vi "QPSK Modulation.vi"(10 "standard deviation":dbl=1.0000000000000002 format="%0.2f", 11 "Sequence Size":i32) -> (1 "Transmitted Signal":waveform(dbl)(graph), 2 "input bits":dbl[](array[numeric]), 3 "Input Graph":dbl[](graph))   [LabVIEW 2026]
panel:
  out "size(s)":i32
  out "Array":dynamicdata[](array[waveform])
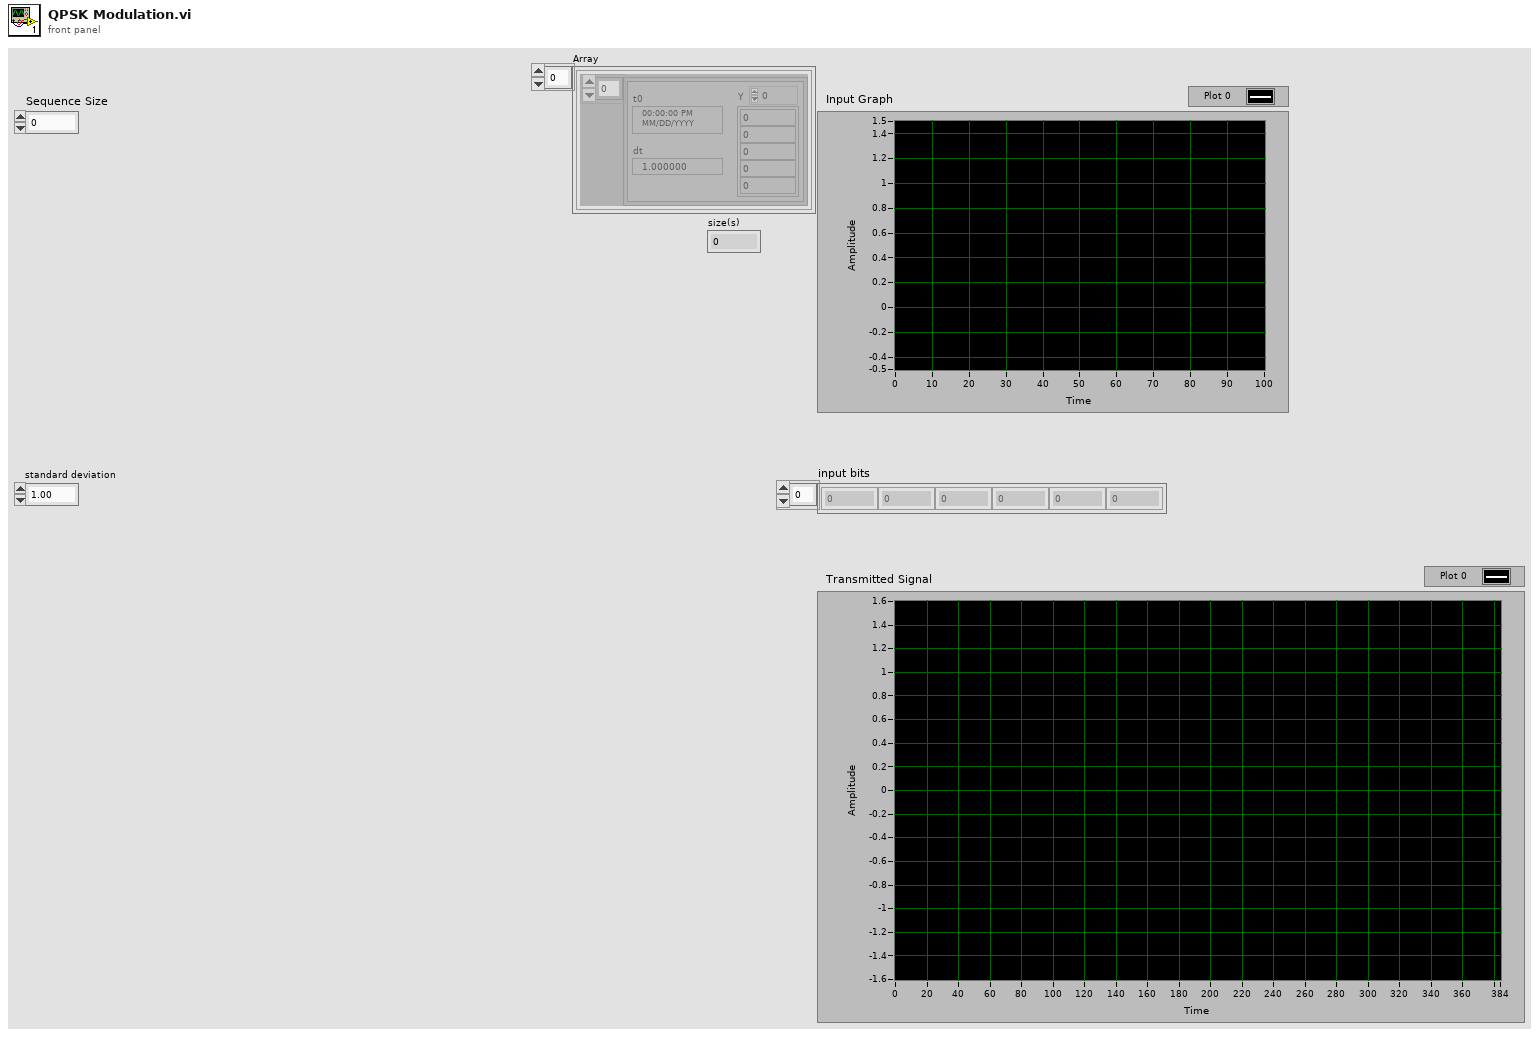
[diagram p1: front panel]
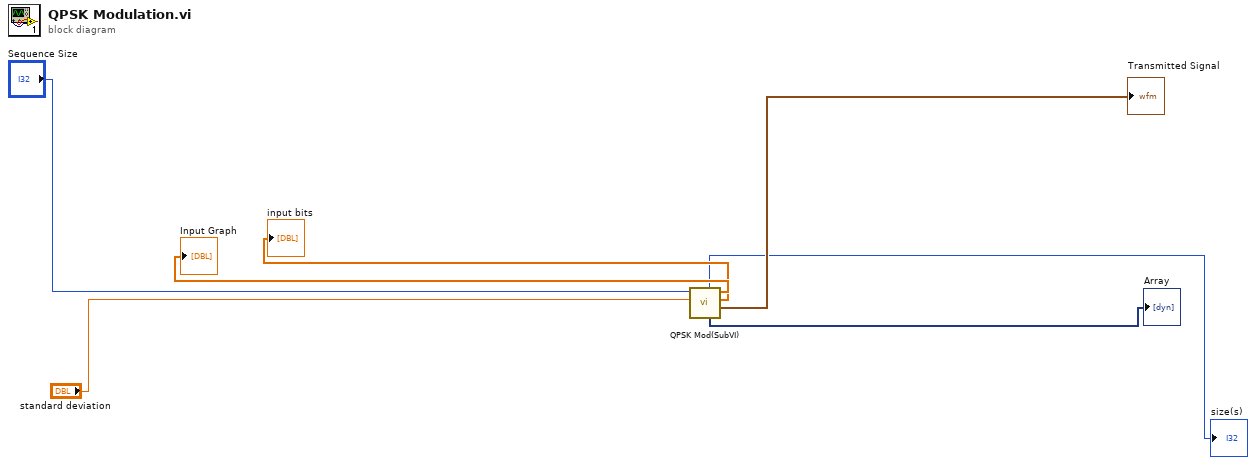
[diagram p0: block diagram]
diagram:
  n1 = call "QPSK Mod(SubVI).vi"("standard deviation"="standard deviation", "Sequence Size"="Sequence Size") -> ("Transmitted Signal"=→"Transmitted Signal":waveform(dbl), "input bits"=→"input bits":dbl[], "Input Graph"=→"Input Graph":dbl[], "Array"=→"Array":dynamicdata[], "size(s)"=→"size(s)":i32)  [unwired: 5 in]
